vi "TCP_WriteRead.vi"(6 "error in (no error)":errorcluster, 8 "data in":string, 9 "connectin ID in":refnum<k5>) -> (0 "error out":errorcluster, 2 "data out":string, 3 "connectin ID out":refnum<k5>)   [LabVIEW 2020]
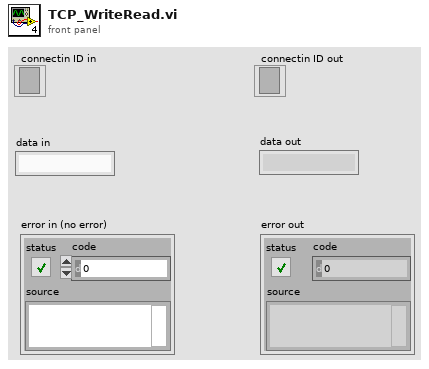
[diagram p1: front panel]
types:
  T1 = enum16{"Standard", "Buffered", "CRLF", "Immediate"}
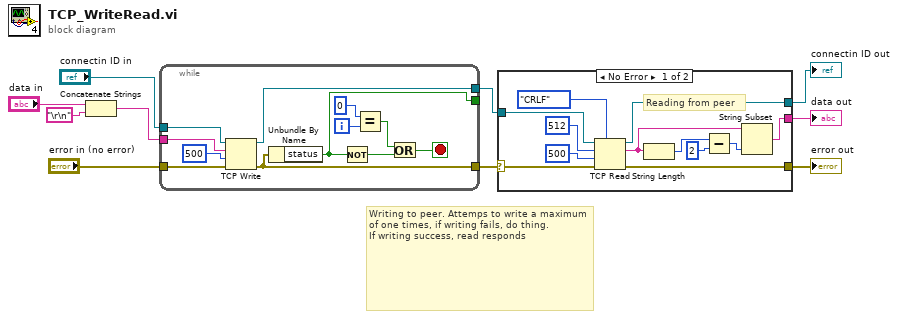
[diagram p0: block diagram]
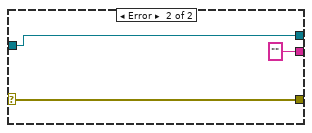
[diagram p2: hidden frame]
diagram:
  # "Writing to peer. Attemps to write a maximum of one times, if writing fails, do thing.\nIf writing success, read responds"
  n1 = Concatenate Strings("data in", "\r\n") -> (w4:string)
  n2 = while {
    tunnel: [w22] -> w8
    tunnel: w4 -> [w21]
    tunnel: "connectin ID in" -> [w20]
    tunnel: [w14] -> _
    tunnel: "error in (no error)" -> [w12]
    tunnel: [w11] -> w1
    i -> [w19]
    stop <- w15 stop-if-true
    n3 = TCP Write(connection ID=w20, data in=w21, error in (no error)=w12, 9:500 ("timeout ms (25000)")) -> (connection ID out=w22:refnum<k5>, error out=w11:errorcluster)  [unwired: 1 out]
    n4 = Unbundle By Name(w11) -> ("status"=w14:bool)
    n5 = Not(x=w14) -> (.not. x?=w16:bool)
    n6 = Equal?(x=0, y=w19) -> (x = y?=w17:bool)
    n7 = Or(x=w17, y=w16) -> (x .or. y?=w15:bool)
  }
  n8 = case shown="No Error" w1 {
    selector: w1 -> [w23 w35]
    tunnel: [w31 "" ("data out")] -> w10
    tunnel: [w28 w37] -> w9
    tunnel: w8 -> [w27 w37]
    tunnel: [w24 w35] -> w2
    frame No Error {
      # "Reading from peer"
      n9 = TCP Read(connection ID=w27, bytes to read=512, error in (no error)=w23, 7:T1."CRLF" ("mode (standard)"), 9:500 ("timeout ms (25000)")) -> (connection ID out=w28:refnum<k5>, data out=w26:string, error out=w24:errorcluster)
      n10 = String Length(string=w26) -> (length=w32:i32)
      n11 = Subtract(x=w32, y=2 ("length (rest)")) -> (x-y=w34:i32)
      n12 = String Subset(string=w26, length (rest)=w34) -> (substring=w31:string)  [unwired: 1 in]
    }
    frame Error {
    }
  }
  "data out" <- w10
  "connectin ID out" <- w9
  "error out" <- w2
